vi "GetOutputChSettings.vi"(8 "error in (no error)":errorcluster, 10 "ChannelName":T1=enum."Trigger", 11 "T560Session in":refnum<class "T560Session.lvclass">) -> (0 "error out":errorcluster, 2 "OutputSettings":T2, 3 "T560Session out":refnum<class "T560Session.lvclass">)   [LabVIEW 2013, in "T560Session.lvclass"]
doc: "Retrive the trigger settings from the Trigger object"
uses:
  T560Session.lvclass
  Common/TypeDefs/ChannelName.ctl
  T560OutputClass/T560Output.lvclass
  T560ChannelClass/T560Channel.lvclass
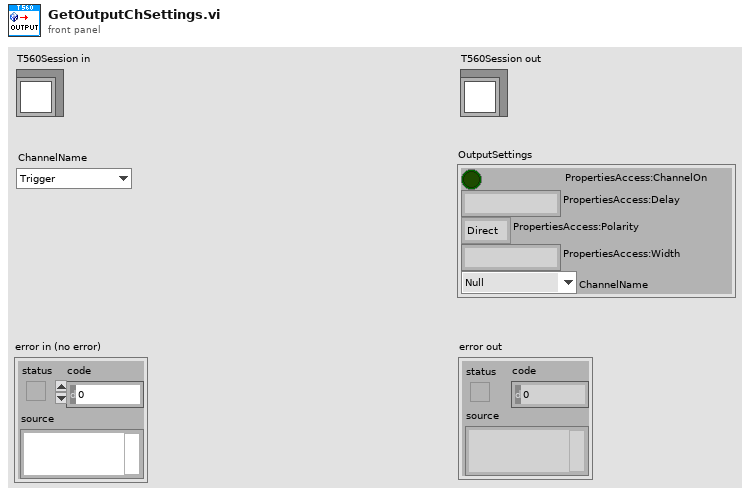
[diagram p1: front panel]
types:
  T1 = typedef "T560Channel.lvclass/ChannelName.ctl" = enum16{"Null", "A", "B", "C", "D", "Trigger"}
  T2 = cluster{"PropertiesAccess:ChannelOn":bool, "PropertiesAccess:Delay":string, "PropertiesAccess:Polarity":enum16{"Direct", "Inverted"}, "PropertiesAccess:Width":string, "ChannelName":T1}
  T3 = typedef "Highlandt564.lvlib/T560Channel.lvclass/ChannelName.ctl" = enum16{"Null", "A", "B", "C", "D", "Trigger"}
  T4 = cluster{"PropertiesAccess:ChannelOn":bool, "PropertiesAccess:Delay":string, "PropertiesAccess:Polarity":enum16{"Direct", "Inverted"}, "PropertiesAccess:Width":string, "ChannelName":T3}
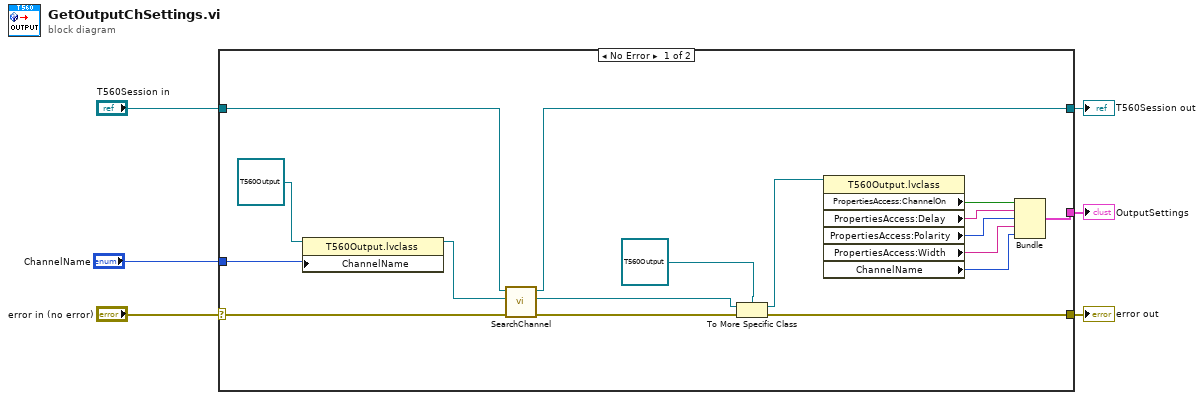
[diagram p0: block diagram]
diagram:
  n1 = case shown="No Error" "error in (no error)" {
    selector: "error in (no error)" -> [w20 w25]
    tunnel: [w18 w25] -> w5
    tunnel: [w22 w24] -> w3
    tunnel: "T560Session in" -> [w23 w24]
    tunnel: [w16 _] -> w1
    tunnel: "ChannelName" -> [w13 _]
    frame No Error {
      n2 = property class="T560Output.lvclass"(reference=refnum<class "T560Output.lvclass"> refnum ("Highlandt564.lvlib:T560Output.lvclass"), "ChannelName"=w13) -> (reference out=w21:refnum<class "T560Output.lvclass">)  [unwired: 1 in, 1 out]
      n3 = call-dynamic "SearchChannel.vi"("error in"=w20, "T560Channel.lvclass"=w21, "T560Session in"=w23) -> ("error out"=w19:errorcluster, "T560Object.lvclass"=w15:refnum<class "T560Channel.lvclass">, "T560Session out"=w22:refnum<class "T560Session.lvclass">)  [unwired: 5 in, 1 out]
      n4 = To More Specific Class(target class=refnum<class "T560Output.lvclass"> refnum ("Highlandt564.lvlib:T560Output.lvclass"), reference=w15, error in=w19) -> (specific class reference=w17:refnum<class "T560Output.lvclass">, error out=w18:errorcluster)
      n5 = property class="T560Output.lvclass"(reference=w17) -> ("PropertiesAccess:ChannelOn"=w11:bool, "PropertiesAccess:Delay"=w10:string, "PropertiesAccess:Polarity"=w9:enum16{"Direct", "Inverted"}, "PropertiesAccess:Width"=w8:string, "ChannelName"=w7:T3)  [unwired: 1 in, 2 out]
      n6 = Bundle("PropertiesAccess:ChannelOn"=w11, "PropertiesAccess:Delay"=w10, "PropertiesAccess:Polarity"=w9, "PropertiesAccess:Width"=w8, "ChannelName"=w7) -> (w16:T4)  [unwired: 1 in]
    }
    frame Error {
    }
  }
  "error out" <- w5
  "T560Session out" <- w3
  "OutputSettings" <- w1
